vi "Controlador_grados_a_pasos.vi"(8 "error in (no error)":errorcluster, 11 "array_grados":i64[][](array[numeric])) -> (0 "error in (no error) 2":errorcluster, 2 "array_pasos":i32[][](array[numeric]))   [LabVIEW 2026]
uses:
  GlobalVariable/Muestreo.vi
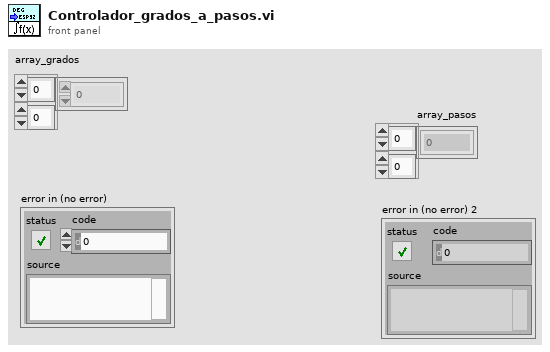
[diagram p1: front panel]
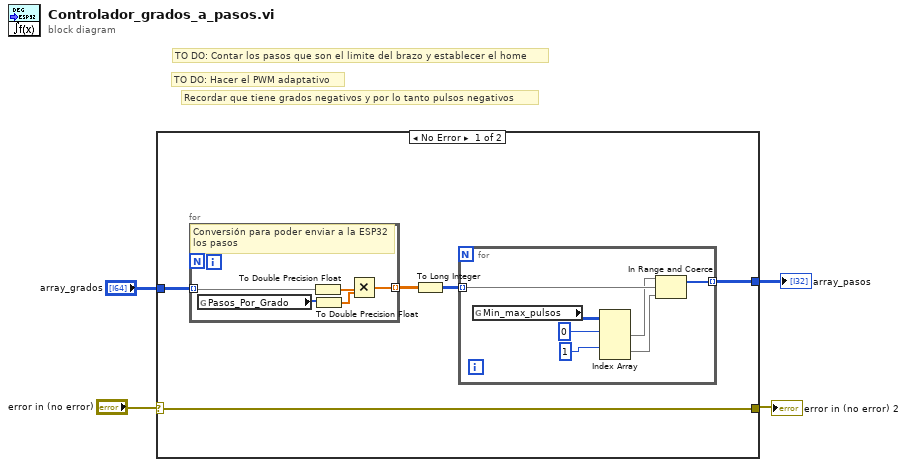
[diagram p0: block diagram]
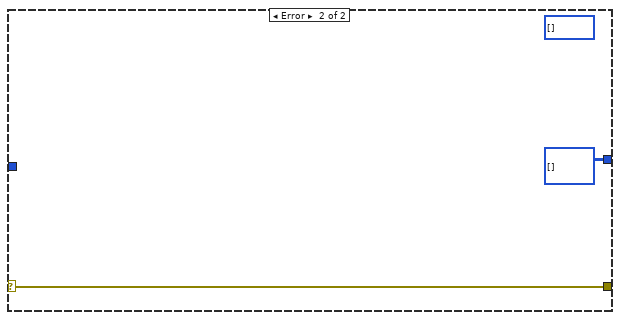
[diagram p2: hidden frame]
diagram:
  # "TO DO: Contar los pasos que son el limite del brazo y establecer el home"
  # "Recordar que tiene grados negativos y por lo tanto pulsos negativos"
  # "TO DO: Hacer el PWM adaptativo"
  n1 = case shown="No Error" "error in (no error)" {
    selector: "error in (no error)" -> [w9 w23]
    tunnel: [w9 w23] -> w3
    tunnel: "array_grados" -> [w6 _]
    tunnel: [w5 i32[][] []] -> w1
    frame No Error {
      n2 = for {
        tunnel: [w18] -> w8 mode=indexing
        tunnel: w6 -> [w17] mode=indexing
        # "Conversión para poder enviar a la ESP32 los pasos"
        n3 = global read "Muestreo.vi" "Pasos_Por_Grado"() -> (w19:i32[])
        n4 = To Double Precision Float(number=w17) -> (double precision float=w21:dbl[])
        n5 = To Double Precision Float(number=w19) -> (double precision float=w20:dbl[])
        n6 = Multiply(x=w21, y=w20) -> (x*y=w18:dbl[])
      }
      n7 = To Long Integer(number=w8) -> (32bit integer=w7:i32[][])
      n8 = for {
        tunnel: w7 -> [w15] mode=indexing
        tunnel: [w10] -> w5 mode=indexing
        n9 = global read "Muestreo.vi" "Min_max_pulsos"() -> (w16:i32[][])
        n10 = Index Array(array=w16, index (row) #1=0 ("disabled index (col)"), index (row) #2=1 ("disabled index (col)")) -> (element #1=w12:i32[], element #2=w11:i32[])  [unwired: 2 in]
        n11 = In Range and Coerce(upper limit=w12, x=w15, lower limit=w11) -> (coerced(x)=w10:i32[])  [unwired: 1 out]
      }
    }
    frame Error {
      (unwired) i32[] []
    }
  }
  "error in (no error) 2" <- w3
  "array_pasos" <- w1
